vi "Calculation steps for full mode (SILAR).vi"(0 "Loop iteration для кол-ва циклов":dbl, 1 "Кол-во жидкости в каждом стакане [мм]":dbl, 2 "Высота стакана [мм]":dbl=81.2, 3 "Высота подложки [мм]":dbl, 4 "Loop iteration для кол-ва используемых растворов":i32, 5 "Loop iteration для кол-ва погружений в каждый стакан":i32) -> (14 "Кол-во шагов до раствора":dbl, 16 "Кол-во шагов из раствора":dbl, 18 "Кол-во шагов над раствором":dbl)   [LabVIEW 2016]
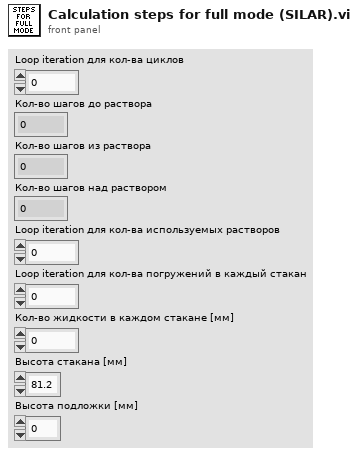
[diagram p1: front panel]
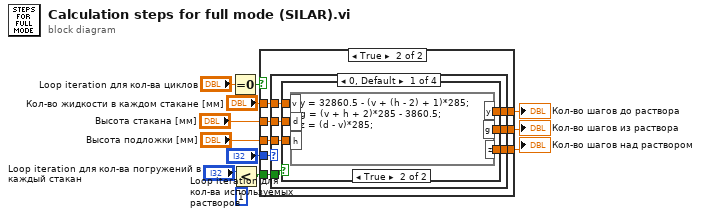
[diagram p0: block diagram]
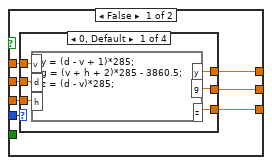
[diagram p2: hidden frame]
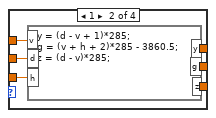
[diagram p3: hidden frame]
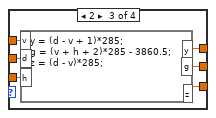
[diagram p4: hidden frame]
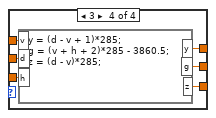
[diagram p5: hidden frame]
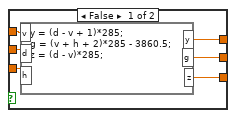
[diagram p6: hidden frame]
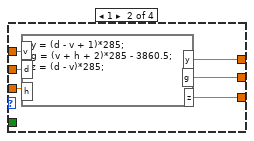
[diagram p7: hidden frame]
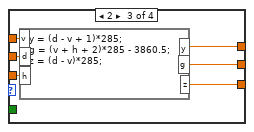
[diagram p8: hidden frame]
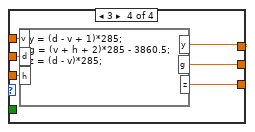
[diagram p9: hidden frame]
diagram:
  n1 = Equal To 0?(x="Loop iteration для кол-ва циклов") -> (x = 0?=w3:bool)
  n2 = Less?(x="Loop iteration для кол-ва погружений в каждый стакан", y=1) -> (x < y?=w11:bool)
  n3 = case shown="True" w3 {
    tunnel: "Кол-во жидкости в каждом стакане [мм]" -> [w19 w51]
    tunnel: "Высота подложки [мм]" -> [w17 w50]
    tunnel: [w15 w49] -> w6
    tunnel: "Loop iteration для кол-ва используемых растворов" -> [w16 w47]
    tunnel: "Высота стакана [мм]" -> [w18 w46]
    tunnel: [w14 w48] -> w4
    tunnel: [w13 w45] -> w5
    tunnel: w11 -> [_ w44]
    frame False {
      n4 = case shown="0, Default" w16 {
        tunnel: w19 -> [w25 w31 w37 w43]
        tunnel: w17 -> [w24 w30 w35 w41]
        tunnel: [w23 w29 w34 w40] -> w15
        tunnel: [w22 w28 w33 w39] -> w14
        tunnel: w18 -> [w21 w27 w36 w42]
        tunnel: [w20 w26 w32 w38] -> w13
        frame 0, Default {
          n5 = formula code="y = (d - v + 1)*285;\ng = (v + h + 2)*285 - 3860.5;\nz = (d - v)*285;"("v"=w25, "h"=w24, "d"=w21) -> ("y"=w23:dbl, "z"=w22:dbl, "g"=w20:dbl)
        }
        frame 1 {
          n6 = formula code="y = (d - v + 1)*285;\ng = (v + h + 2)*285 - 3860.5;\nz = (d - v)*285;"("v"=w31, "h"=w30, "d"=w27) -> ("y"=w29:dbl, "z"=w28:dbl, "g"=w26:dbl)
        }
        frame 2 {
          n7 = formula code="y = (d - v + 1)*285;\ng = (v + h + 2)*285 - 3860.5;\nz = (d - v)*285;"("v"=w37, "h"=w35, "d"=w36) -> ("y"=w34:dbl, "z"=w33:dbl, "g"=w32:dbl)
        }
        frame 3 {
          n8 = formula code="y = (d - v + 1)*285;\ng = (v + h + 2)*285 - 3860.5;\nz = (d - v)*285;"("v"=w43, "h"=w41, "d"=w42) -> ("y"=w40:dbl, "z"=w39:dbl, "g"=w38:dbl)
        }
      }
    }
    frame True {
      n9 = case shown="0, Default" w47 {
        tunnel: w51 -> [w58 w76 w82 w88]
        tunnel: w50 -> [w57 w75 w80 w86]
        tunnel: [w56 w74 w79 w85] -> w49
        tunnel: [w55 w73 w78 w84] -> w48
        tunnel: w46 -> [w52 w72 w81 w87]
        tunnel: [w54 w71 w77 w83] -> w45
        tunnel: w44 -> [w53 _ _ _]
        frame 0, Default {
          n10 = case shown="True" w53 {
            tunnel: w58 -> [w64 w70]
            tunnel: w57 -> [w62 w69]
            tunnel: [w61 w68] -> w56
            tunnel: [w59 w67] -> w55
            tunnel: w52 -> [w63 w66]
            tunnel: [w60 w65] -> w54
            frame False {
              n11 = formula code="y = (d - v + 1)*285;\ng = (v + h + 2)*285 - 3860.5;\nz = (d - v)*285;"("v"=w64, "h"=w62, "d"=w63) -> ("y"=w61:dbl, "z"=w59:dbl, "g"=w60:dbl)
            }
            frame True {
              n12 = formula code="y = 32860.5 - (v + (h - 2) + 1)*285;\ng = (v + h + 2)*285 - 3860.5;\nz = (d - v)*285;"("v"=w70, "h"=w69, "d"=w66) -> ("y"=w68:dbl, "z"=w67:dbl, "g"=w65:dbl)
            }
          }
        }
        frame 1 {
          n13 = formula code="y = (d - v + 1)*285;\ng = (v + h + 2)*285 - 3860.5;\nz = (d - v)*285;"("v"=w76, "h"=w75, "d"=w72) -> ("y"=w74:dbl, "z"=w73:dbl, "g"=w71:dbl)
        }
        frame 2 {
          n14 = formula code="y = (d - v + 1)*285;\ng = (v + h + 2)*285 - 3860.5;\nz = (d - v)*285;"("v"=w82, "h"=w80, "d"=w81) -> ("y"=w79:dbl, "z"=w78:dbl, "g"=w77:dbl)
        }
        frame 3 {
          n15 = formula code="y = (d - v + 1)*285;\ng = (v + h + 2)*285 - 3860.5;\nz = (d - v)*285;"("v"=w88, "h"=w86, "d"=w87) -> ("y"=w85:dbl, "z"=w84:dbl, "g"=w83:dbl)
        }
      }
    }
  }
  "Кол-во шагов до раствора" <- w6
  "Кол-во шагов из раствора" <- w5
  "Кол-во шагов над раствором" <- w4
